vi "Result.vi"(8 "error in (no error)":errorcluster, 10 "Results":T1={"Name"="", "Message"="", "Description"="", "Status"=enum."Passed", "Result Type"=enum."Test Suite", "Execution Time"=0.0}, 11 "Result Model In":refnum<class "Result Model.lvclass">) -> (0 "error out":errorcluster, 3 "Result Model Out":refnum<class "Result Model.lvclass">)   [LabVIEW 2020, in "Result Model.lvclass"]
uses:
  Result Model.lvclass
  Core/Result/Result.ctl
  Core/Result/Status.ctl
  Core/Result/Type.ctl
  Core/Result/Result.lvlib
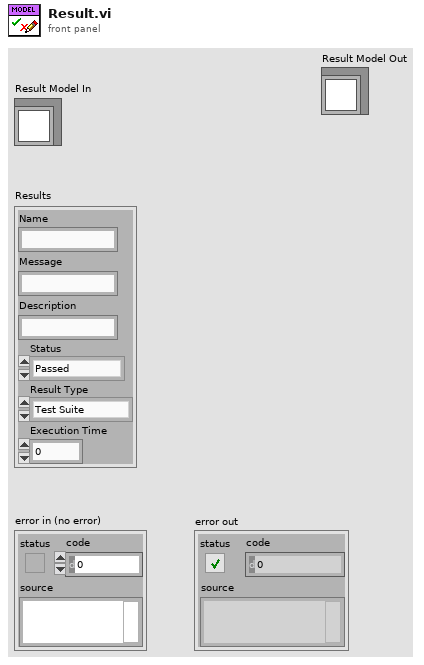
[diagram p1: front panel]
types:
  T1 = typedef "Result.lvlib/Result.ctl" = cluster{"Name":string, "Message":string, "Description":string, "Status":T2, "Result Type":T3, "Execution Time":dbl}
  T2 = typedef "Result.lvlib/Status.ctl" = enum16{"", "Passed", "Failed", "Error", "Skipped", "Setup Error", "Broken", "Teardown Error"}
  T3 = typedef "Result.lvlib/Type.ctl" = enum16{"Test Case", "Test Suite", "Test Run", "Pass", "Fail", "Skip", "Pass if", "Fail if", "Pass if Error", "Fail if Error", "Pass if Equal", "Fail if Equal"}
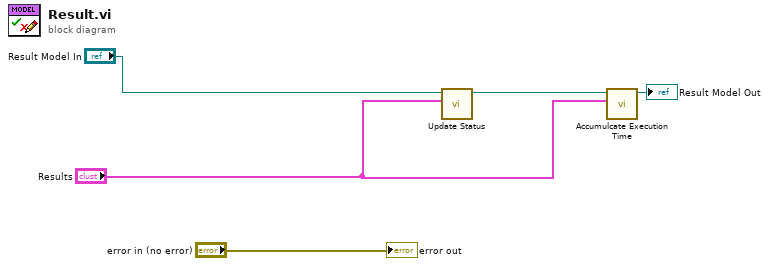
[diagram p0: block diagram]
diagram:
  n1 = call "Update Status.vi"("Result"="Results", "Result Model In"="Result Model In") -> ("Result Model Out"=w2:refnum<class "Result Model.lvclass">)  [unwired: 9 in]
  n2 = call "Accumulcate Execution Time.vi"("Result"="Results", "Result Model In"=w2) -> ("Result Model Out"=→"Result Model Out":refnum<class "Result Model.lvclass">)  [unwired: 9 in]
  "error out" <- "error in (no error)"
